vi "Replace Named Format Specifier Test.vi"() -> ()   [LabVIEW 2018]
uses:
  api/configuration/formatters/format_string_formatter/Format String.lvclass
panel:
  out "error out":errorcluster
  out "resulting string":string="hello, world\nFFFFFFFFFFFFFE5B\n1777777777777777777133\n1111111111111111111111111111111111111111111111111111111001011011\n-421\n0\n-420.690000\n-4.206900E+2\n-420.690000\n-420.690000\npath\\to\\nowhere\n123645789\n10:20:15.526 PM 1/23/2025\nthird\n2\ngood to be here\n1589624.000000"
  in  "format string":string="%{str}$s\n%{dbl}$x\n%{dbl}$o\n%{dbl}$b\n%{dbl}$d\n%{dbl}$u\n%{dbl}$f\n%{dbl}$e\n%{dbl}$g\n%{dbl}$p\n%{path}$s\n%{i32}$d\n%{timestamp}$T\n%{enum}$s\n%{enum}$d\n%{sub.quote}$s\n%{sub.val}$f"
  in  "cluster":T1={"str"="hello, world", "dbl"=-420.69, "path"=path "path/to/nowhere", "i32"=123645789, "timestamp"=timestamp(3820544415.5264506 s since 1904-01-01), "enum"=enum."third", "sub"={"quote"="good to be here", "val"=1589624.0}, "name.with.dots"=15987, "name\\with\\slashes"=7862199, "name.with\\both"=16874654, "fxp"=144984.0}
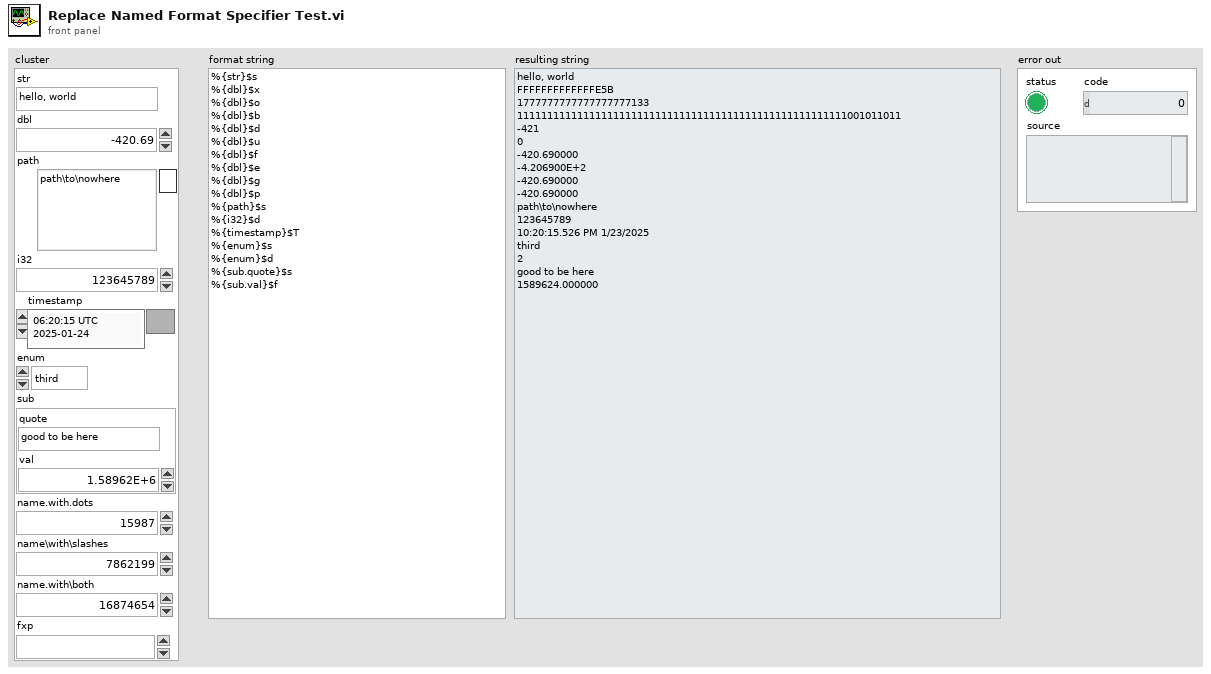
[diagram p1: front panel]
types:
  T1 = cluster{"str":string, "dbl":dbl, "path":path, "i32":i32, "timestamp":timestamp, "enum":enum16{"first", "second", "third"}, "sub":cluster{"quote":string, "val":dbl}, "name.with.dots":i32, "name\\with\\slashes":i32, "name.with\\both":i32, "fxp":fxp<+/-,64,32>}
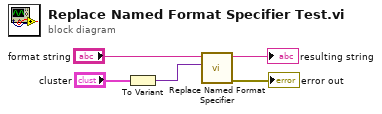
[diagram p0: block diagram]
diagram:
  n1 = To Variant(anything="cluster") -> (Variant=w4:variant)
  n2 = call "Replace Named Format Specifier.vi"("data"=w4, "format string"="format string") -> ("error out"=→"error out":errorcluster, "resulting string"=→"resulting string":string)  [unwired: 8 in]
